vi "Laser Firing FGV.vi"(8 "error in (no error)":errorcluster, 10 "Laser Firing":bool, 11 "Action":T1) -> (0 "error out":errorcluster, 2 "Laser Firing":bool)   [LabVIEW 2022 SP3, in "Test Station SIM Laser Driver.lvclass"]
uses:
  Test Station SIM Laser Driver.lvclass
  Test Station SIM Laser Driver.lvclass/Test Station SIM Laser Driver.ctl
  Action.ctl
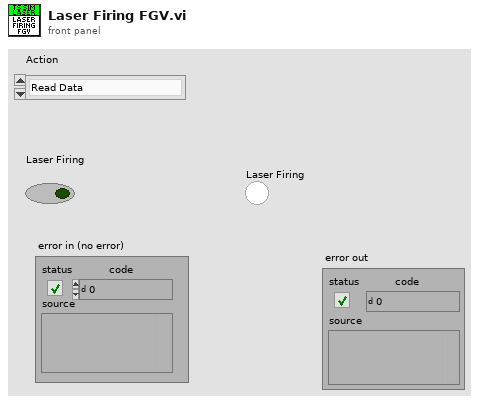
[diagram p1: front panel]
types:
  T1 = typedef "Test Station SIM Laser Driver.lvclass/Action.ctl" = enum16{"Read Data", "Set Data"}
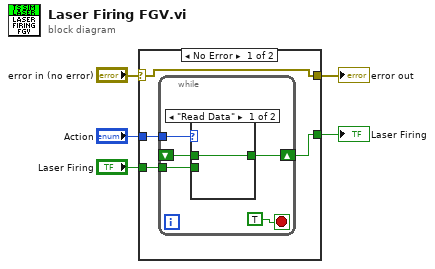
[diagram p0: block diagram]
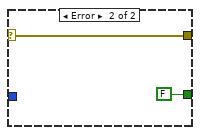
[diagram p3: hidden frame]
diagram:
  n1 = case shown="No Error" "error in (no error)" {
    selector: "error in (no error)" -> [w6 w18]
    tunnel: "Action" -> [w9 _]
    tunnel: "Laser Firing" -> [w8 _]
    tunnel: [w7 FALSE ("Laser Firing")] -> w3
    tunnel: [w6 w18] -> w1
    frame No Error {
      n2 = while {
        tunnel: w9 -> [w13]
        tunnel: w8 -> [w12]
        shift-right: [w11] -> w7
        shift-left: _ -> [w10]
        stop <- TRUE stop-if-true
        n3 = case shown="\"Read Data\"" w13 {
          tunnel: w12 -> [_ w16]
          tunnel: [w15 w16] -> w11
          tunnel: w10 -> [w15 _]
          frame "Read Data" {
          }
          frame "Set Data" {
          }
        }
      }
    }
    frame Error {
    }
  }
  "Laser Firing" <- w3
  "error out" <- w1
